vi "Max logic.vi"() -> ()   [LabVIEW 2019]
panel:
  out "Reverse":bool
  out "Max Val":sgl
  out "stop":bool
  out "Iteration (i-1)":sgl
  out "Iteration (i-2)":sgl
  out "Current Val":sgl
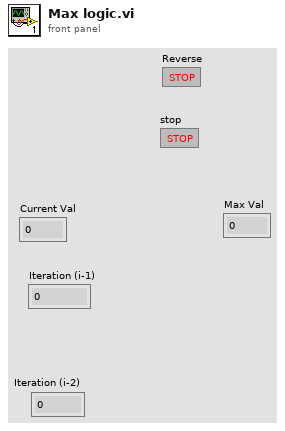
[diagram p1: front panel]
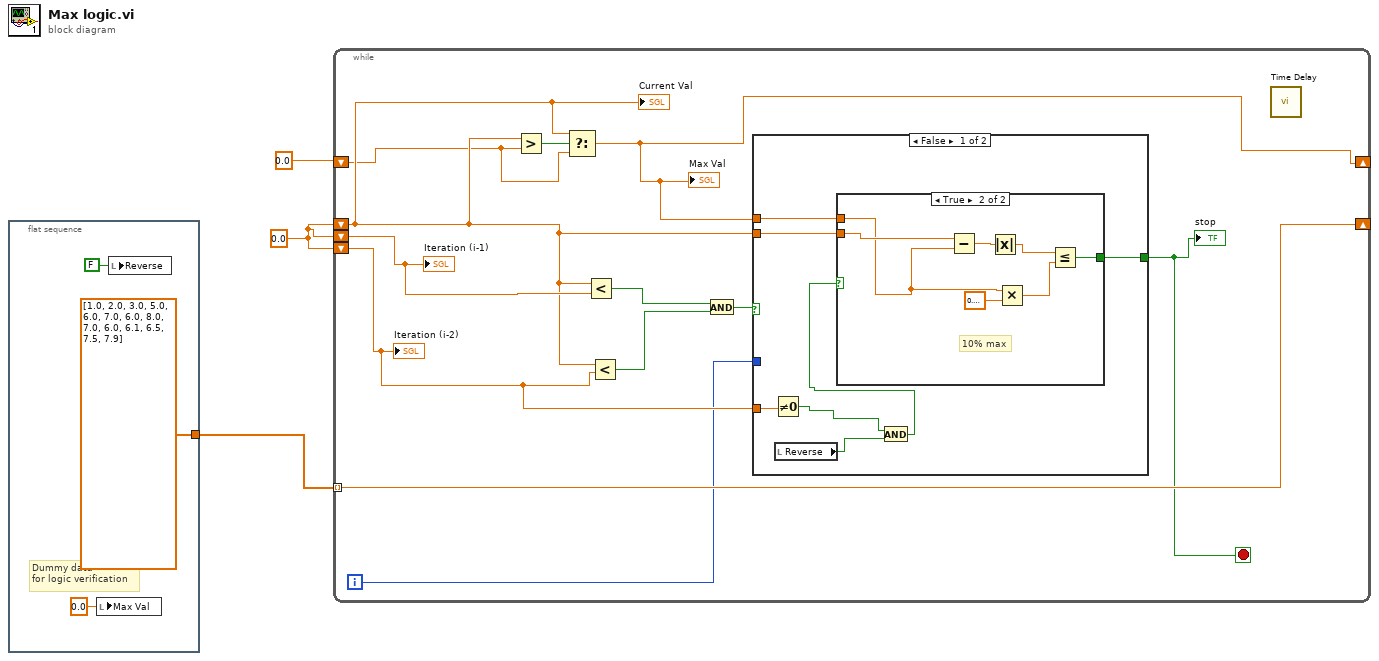
[diagram p0: block diagram]
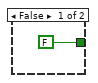
[diagram p2: hidden frame]
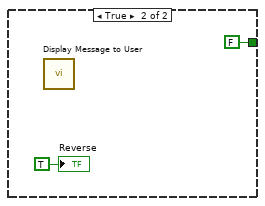
[diagram p3: hidden frame]
diagram:
  w3 = sgl 0.0
  n1 = flat-sequence {
    tunnel: [dbl[] [1.0, 2.0, 3.0, 5.0, 6.0, 7.0, 6.0, 8.0, 7.0, 6.0, 6.1, 6.5, 7.5, 7.9]] -> w1
    frame #0 {
      # "Dummy data\nfor logic verification"
      n2 = local write "Max Val"(sgl 0.0 ("Max Val")) -> ()
      n3 = local write "Reverse"(FALSE ("Reverse")) -> ()
    }
  }
  n4 = while {
    shift-right: [w14] -> _
    shift-left: w3 -> [w9]
    shift-left: w3 -> [w18]
    shift-left: w3 -> [w13]
    tunnel: w1 -> [w14] mode=indexing
    shift-right: [w7] -> _
    shift-left: sgl 0.0 -> [w8]
    i -> [w11]
    stop <- w12 stop-if-true
    n5 = Greater?(x=w9, y=w8) -> (0:w10:bool)
    n6 = Select(t=w9, s=w10, f=w8) -> (s? t:f=w7:dbl)
    "Max Val" <- w7
    n7 = Less?(x=w9, y=w18) -> (x < y?=w17:bool)
    n8 = Less?(x=w9, y=w13) -> (x < y?=w16:bool)
    n9 = And(x=w17, y=w16) -> (x .and. y?=w15:bool)
    n10 = case shown="False" w15 {
      tunnel: w13 -> [w23 _]
      tunnel: w9 -> [w25 _]
      tunnel: [w24 FALSE] -> w12
      tunnel: w11 -> [_ _]
      tunnel: w7 -> [w22 _]
      frame False {
        n11 = Not Equal To 0?(x=w23) -> (x != 0?=w20:bool)
        n12 = local read "Reverse"() -> (w21:bool)
        n13 = And(x=w20, y=w21) -> (x .and. y?=w19:bool)
        n14 = case shown="True" w19 {
          tunnel: w25 -> [_ w33]
          tunnel: [FALSE w30] -> w24
          tunnel: w22 -> [_ w27]
          frame False {
          }
          frame True {
            # "10% max"
            n15 = Subtract(x=w33, y=w27) -> (x-y=w32:dbl)
            n16 = Absolute Value(x=w32) -> (abs(x)=w28:dbl)
            n17 = Multiply(x=w27, y=sgl 0.1) -> (x*y=w29:dbl)
            n18 = Less Or Equal?(x=w28, y=w29) -> (x <= y?=w30:bool)
          }
        }
      }
      frame True {
        n19 = call "Display Message to User"() -> ()  [unwired: 10 in, 2 out]
        "Reverse" <- TRUE ("Reverse")
      }
    }
    "stop" <- w12
    n20 = call "Time Delay"() -> ()  [unwired: 11 in, 1 out]
    "Current Val" <- w9
    "Iteration (i-2)" <- w13
    "Iteration (i-1)" <- w18
  }
